vi "ROSmsg_getTermRef.vi"(9 "Name":string, 11 "SubVI Refnum":refnum<vi>) -> (1 "Term Refnum":refnum<vi>, 2 "Exists?":bool, 3 "SubVI Refnum 2":refnum<vi>)   [LabVIEW 2012]
doc: "Returns a reference to the specified Terminal"
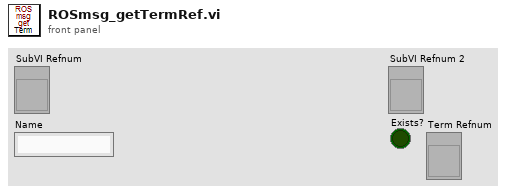
[diagram p1: front panel]
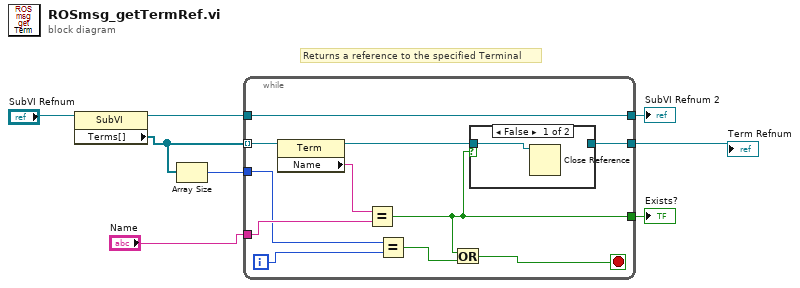
[diagram p0: block diagram]
diagram:
  # "Returns a reference to the specified Terminal"
  n1 = property class="SubVI"(reference="SubVI Refnum") -> (reference out=w4:refnum<vi>, "Terms[]"=w6:refnum<vi>[])  [unwired: 1 in, 1 out]
  n2 = Array Size(array=w6) -> (size(s)=w5:i32)
  n3 = while {
    tunnel: w6 -> [w19] mode=indexing
    tunnel: "Name" -> [w17]
    tunnel: w5 -> [w15]
    tunnel: w4 -> [w12]
    tunnel: [w12] -> w3
    tunnel: [w10] -> w2
    tunnel: [w9] -> w1
    i -> [w16]
    stop <- w13 stop-if-true
    n4 = property class="Term"(reference=w19) -> (reference out=w11:refnum<vi>, "Name"=w18:string)  [unwired: 1 in, 1 out]
    n5 = Equal?(x=w18, y=w17) -> (x = y?=w10:bool)
    n6 = Equal?(x=w15, y=w16) -> (x = y?=w14:bool)
    n7 = Or(x=w10, y=w14) -> (x .or. y?=w13:bool)
    n8 = case shown="False" w10 {
      tunnel: w11 -> [w20 w21]
      tunnel: [_ w21] -> w9
      frame False {
        n9 = Close Reference(reference=w20) -> ()  [unwired: 1 in, 1 out]
      }
      frame True {
      }
    }
  }
  "SubVI Refnum 2" <- w3
  "Exists?" <- w2
  "Term Refnum" <- w1
